vi "Init - Preallocate.vi"(5 "I/O timing (ns)":T1, 7 "Samples to allocate":i32, 8 "error in (no error)":errorcluster, 9 "Default transition action":T2, 10 "Sample rate":dbl format="%#_6p", 11 "I2C timing (ns)":T3 {"fSCL" format="%#_6p"}) -> (0 "error out":errorcluster, 1 "Coerced I/O timing (ns)":T1, 2 "Coerced I2C timing (ns)":T3 {"fSCL" format="%#_6p"}, 3 "I2C waveform info":T4)   [LabVIEW 2009, in "IDW.lvlib"]
doc: "Initializes an I2C waveform. Timing parameters are coerced to edges at the given sample rate. The coerced values are output from the VI.\n\nThis is a polymorphic instance of the <b>Init</b> VI. In this instance, buffers are preallocated in memory for the I2C waveform generation operations."
uses:
  IDW.lvlib
  _Typedefs/Waveform info.ctl
  _Typedefs/Timing - ticks.ctl
  _Typedefs/Default transition action.ctl
  _Typedefs/Bit type.ctl
  _Typedefs/Timing - ns.ctl
  _Typedefs/IO timing - ns.ctl
panel:
  # "30-70% rise requested instead of 0-30% so scope measurement is more accurate."
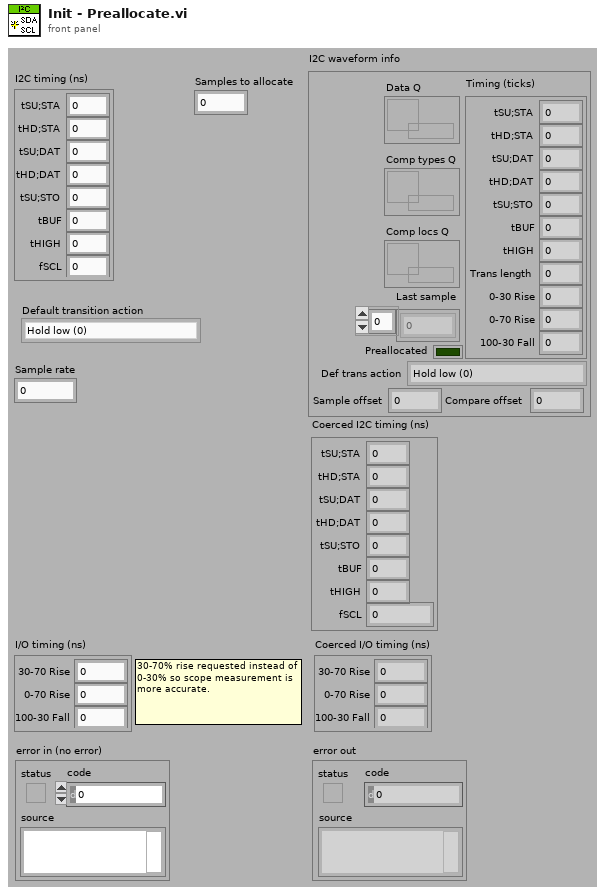
[diagram p1: front panel]
types:
  T1 = typedef "IDW.lvlib/IO timing - ns.ctl" = cluster{"30-70 Rise":dbl, "0-70 Rise":dbl, "100-30 Fall":dbl}
  T2 = typedef "IDW.lvlib/Default transition action.ctl" = enum16{"Hold low (0)", "Release (Z)", "Set up next value", "Hold previous value", "Preserve tHD;DAT and tSU;DAT"}
  T3 = typedef "IDW.lvlib/Timing - ns.ctl" = cluster{"tSU;STA":i32, "tHD;STA":i32, "tSU;DAT":i32, "tHD;DAT":i32, "tSU;STO":i32, "tBUF":i32, "tHIGH":i32, "fSCL":dbl}
  T4 = typedef "IDW.lvlib/Waveform info.ctl" = cluster{"Last sample":u8[], "Sample offset":u64, "Compare offset":u64, "Timing (ticks)":T5, "Preallocated":bool, "Def trans action":T2, "Data Q":refnum<queue>, "Comp types Q":refnum<queue>, "Comp locs Q":refnum<queue>}
  T5 = typedef "IDW.lvlib/Timing - ticks.ctl" = cluster{"tSU;STA":i32, "tHD;STA":i32, "tSU;DAT":i32, "tHD;DAT":i32, "tSU;STO":i32, "tBUF":i32, "tHIGH":i32, "Trans length":i32, "0-30 Rise":i32, "0-70 Rise":i32, "100-30 Fall":i32}
  T6 = typedef "IDW.lvlib/Bit type.ctl" = enum16{"ACK", "Data"}
  T7 = cluster{"tSU;STA":dbl, "tHD;STA":dbl, "tSU;DAT":dbl, "tHD;DAT":dbl, "tSU;STO":dbl, "tBUF":dbl, "tHIGH":dbl, "fSCL":dbl}
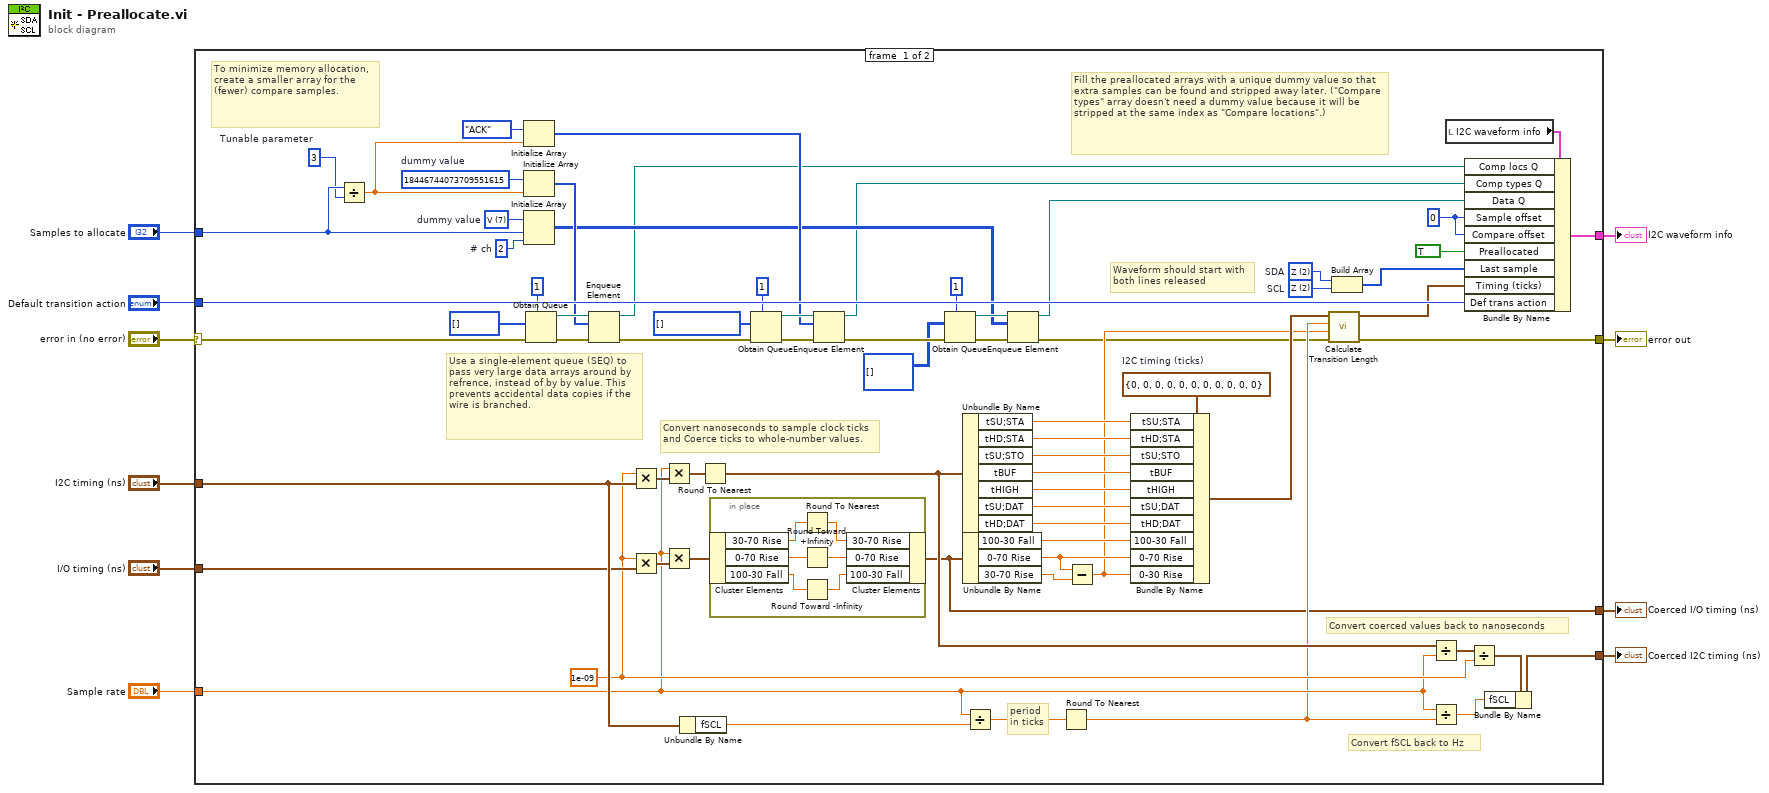
[diagram p0: block diagram]
diagram:
  n1 = case shown="No Error" "error in (no error)" {
    selector: "error in (no error)" -> [w32 w88]
    tunnel: [w77 _] -> w6
    tunnel: "I2C timing (ns)" -> [w60 w87]
    tunnel: "Sample rate" -> [w40 _]
    tunnel: [w39 w88] -> w8
    tunnel: "Samples to allocate" -> [w57 _]
    tunnel: [w62 w87] -> w4
    tunnel: "I/O timing (ns)" -> [w50 w86]
    tunnel: "Default transition action" -> [w52 _]
    tunnel: [w33 w86] -> w1
    frame #0 {
      w22 = T6[] [] items=["ACK", "Data"] ("initialized array")
      w42 = T5 {"tSU;STA"=0, "tHD;STA"=0, "tSU;DAT"=0, "tHD;DAT"=0, "tSU;STO"=0, "tBUF"=0, "tHIGH"=0, "Trans length"=0, "0-30 Rise"=0, "0-70 Rise"=0, "100-30 Fall"=0}  # I2C timing (ticks)
      w55 = u64 18446744073709551615  # dummy value
      w58 = u64 0 ("Offset")
      w72 = u8 7 items=["0", "1", "Z", "L", "H", "X", "T", "V"]  # dummy value
      w49 = 1e-09
      w79 = u8 2 items=["0", "1", "Z", "L", "H", "X", "T", "V"]  # SCL
      w78 = u8 2 items=["0", "1", "Z", "L", "H", "X", "T", "V"]  # SDA
      w56 = 3  # Tunable parameter
      w71 = 2  # # ch
      # "Use a single-element queue (SEQ) to pass very large data arrays around by refrence, instead of by by value. This prevents accidental data copies if the wire is branched."
      # "Convert fSCL back to Hz"
      # "To minimize memory allocation, create a smaller array for the (fewer) compare samples."
      # "period\nin ticks"
      # "Fill the preallocated arrays with a unique dummy value so that extra samples can be found and stripped away later. (\"Compare types\" array doesn't need a dummy value because it will be stripped at the same index as \"Compare locations\".)"
      # "Waveform should start with  both lines released"
      # "Convert coerced values back to nanoseconds"
      # "Convert nanoseconds to sample clock ticks and Coerce ticks to whole-number values."
      n2 = Divide(x=w57, y=w56) -> (x/y=w54:dbl)
      n3 = Initialize Array(Bit_type."ACK" ("Compare type"), w54) -> (w21:T6[])
      n4 = Initialize Array(w55, w54) -> (w29:u64[])
      n5 = Initialize Array(w72, w57, w71) -> (w15:u8[][])
      n6 = Obtain Queue(max queue size (-1, unlimited)=1, element data type=u64[] [] ("initialized array"), error in (no error)=w32) -> (queue out=w30:refnum<queue>, error out=w31:errorcluster)  [unwired: 2 in, 1 out]
      n7 = Enqueue Element(queue=w30, element=w29, error in (no error)=w31) -> (queue out=w13:refnum<queue>, error out=w23:errorcluster)  [unwired: 1 in, 1 out]
      n8 = Multiply(x=w49, y=w60) -> (x*y=w74:T7)
      n9 = Multiply(x=w49, y=w50) -> (x*y=w51:T1)
      n10 = Multiply(x=w40, y=w74) -> (x*y=w61:T7)
      n11 = Multiply(x=w40, y=w51) -> (x*y=w34:T1)
      n12 = Unbundle By Name(w60) -> ("fSCL"=w65:dbl)
      n13 = Round To Nearest(number=w61) -> (nearest integer value=w41:T7)
      n14 = in-place {
        n15 = in-place-cluster #1(w34) -> ("30-70 Rise"=w81:dbl, "0-70 Rise"=w83:dbl, "100-30 Fall"=w85:dbl)
        n16 = Round To Nearest(number=w81) -> (nearest integer value=w80:dbl)
        n17 = Round Toward +Infinity(x=w83) -> (ceil(x): smallest int >= x=w82:dbl)
        n18 = Round Toward -Infinity(1:w85) -> (0:w84:dbl)
        n19 = in-place-cluster #1("30-70 Rise"=w80, "0-70 Rise"=w82, "100-30 Fall"=w84) -> (w33:T1)
      }
      n20 = Obtain Queue(max queue size (-1, unlimited)=1, element data type=w22, error in (no error)=w23) -> (queue out=w25:refnum<queue>, error out=w24:errorcluster)  [unwired: 2 in, 1 out]
      n21 = Enqueue Element(queue=w25, element=w21, error in (no error)=w24) -> (queue out=w12:refnum<queue>, error out=w17:errorcluster)  [unwired: 1 in, 1 out]
      n22 = Obtain Queue(max queue size (-1, unlimited)=1, element data type=u8[][] [] ("initialized array"), error in (no error)=w17) -> (queue out=w19:refnum<queue>, error out=w20:errorcluster)  [unwired: 2 in, 1 out]
      n23 = Unbundle By Name(w41) -> ("tSU;STA"=w66:dbl, "tHD;STA"=w67:dbl, "tSU;STO"=w68:dbl, "tBUF"=w69:dbl, "tHIGH"=w47:dbl, "tSU;DAT"=w46:dbl, "tHD;DAT"=w45:dbl)
      n24 = Unbundle By Name(w33) -> ("100-30 Fall"=w44:dbl, "0-70 Rise"=w43:dbl, "30-70 Rise"=w48:dbl)
      n25 = Divide(x=w40, y=w65) -> (x/y=w64:dbl)
      n26 = Enqueue Element(queue=w19, element=w15, error in (no error)=w20) -> (queue out=w11:refnum<queue>, error out=w14:errorcluster)  [unwired: 1 in, 1 out]
      n27 = Round To Nearest(number=w64) -> (nearest integer value=w36:dbl)
      n28 = Subtract(x=w43, y=w48) -> (x-y=w35:dbl)
      n29 = Bundle By Name(cluster=w42, "tSU;STA"=w66, "tHD;STA"=w67, "tSU;STO"=w68, "tBUF"=w69, "tHIGH"=w47, "tSU;DAT"=w46, "tHD;DAT"=w45, "100-30 Fall"=w44, "0-70 Rise"=w43, "0-30 Rise"=w35) -> (w38:T5)
      n30 = call "Calculate Transition Length.vi"("error in (no error)"=w14, "30-70 Rise"=w35, "1/ fSCL"=w36, "I2C timing (ticks)"=w38) -> ("error out"=w39:errorcluster, "I2C timing (ticks) out"=w37:T5)  [unwired: 6 in]
      n31 = Build Array(w78, w79) -> (w75:u8[])
      n32 = Divide(x=w41, y=w40) -> (x/y=w73:T7)
      n33 = Divide(x=w40, y=w36) -> (x/y=w59:dbl)
      n34 = local read "I2C waveform info"() -> (w76:T4)
      n35 = Bundle By Name(cluster=w76, "Comp locs Q"=w13, "Comp types Q"=w12, "Data Q"=w11, "Sample offset"=w58, "Compare offset"=w58, "Preallocated"=TRUE, "Last sample"=w75, "Timing (ticks)"=w37, "Def trans action"=w52) -> (w77:T4)
      n36 = Divide(x=w73, y=w49) -> (x/y=w63:T7)
      n37 = Bundle By Name(cluster=w63, "fSCL"=w59) -> (w62:T7)
    }
    frame #1 {
    }
  }
  "error out" <- w8
  "I2C waveform info" <- w6
  "Coerced I2C timing (ns)" <- w4
  "Coerced I/O timing (ns)" <- w1
